vi "decode_image.vi"(4 "width":i32, 6 "heigth":i32, 8 "Color":bool, 9 "M":i32, 10 "max":i16, 11 "Array":u16[](array[numeric])) -> (0 "error out":errorcluster, 3 "image out":T1(plugin-control))   [LabVIEW 2017]
panel:
  out "size(s) 2":i32
  out "size(s)":i32
  out "Array 2":i32[](array[numeric])
  out "x/y 3":dbl
  out "x/y":dbl
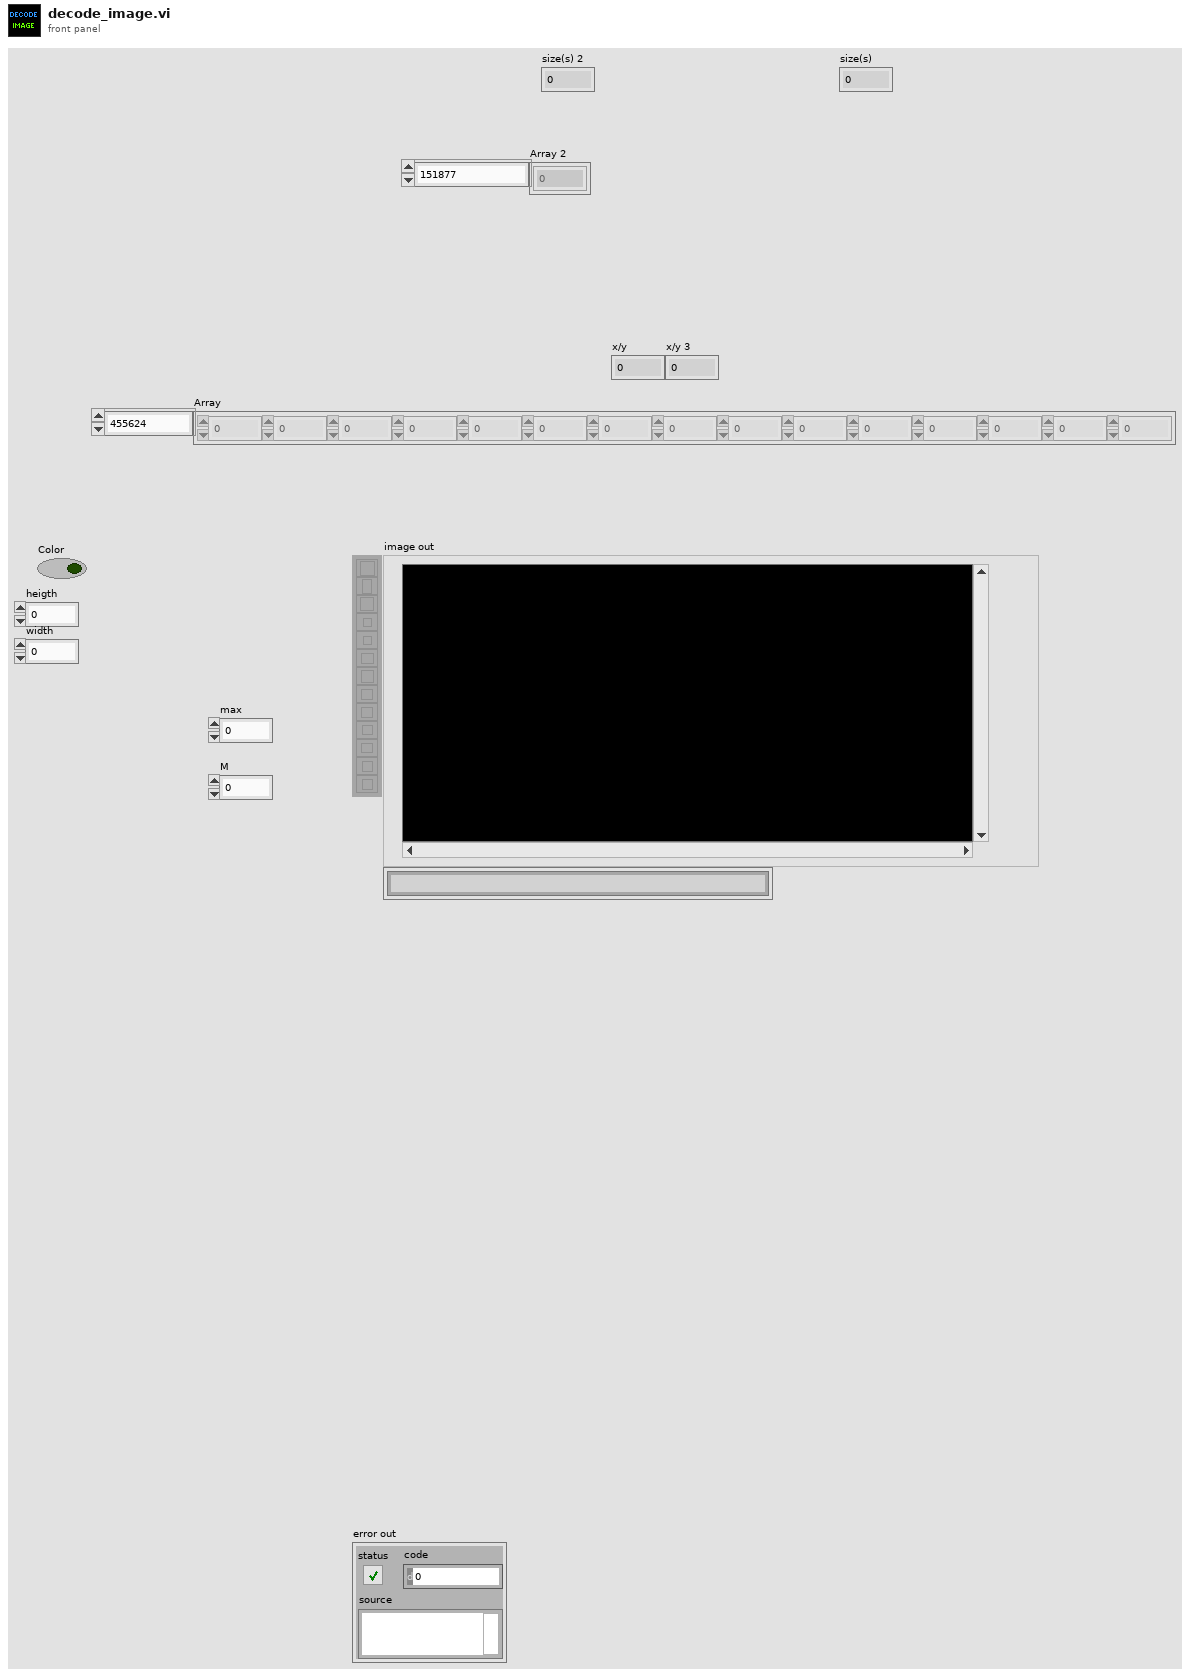
[diagram p1: front panel]
types:
  T1 = typedef "IMAQ Image.ctl" = refnum<image>
  T2 = typedef "Image Type" = u32
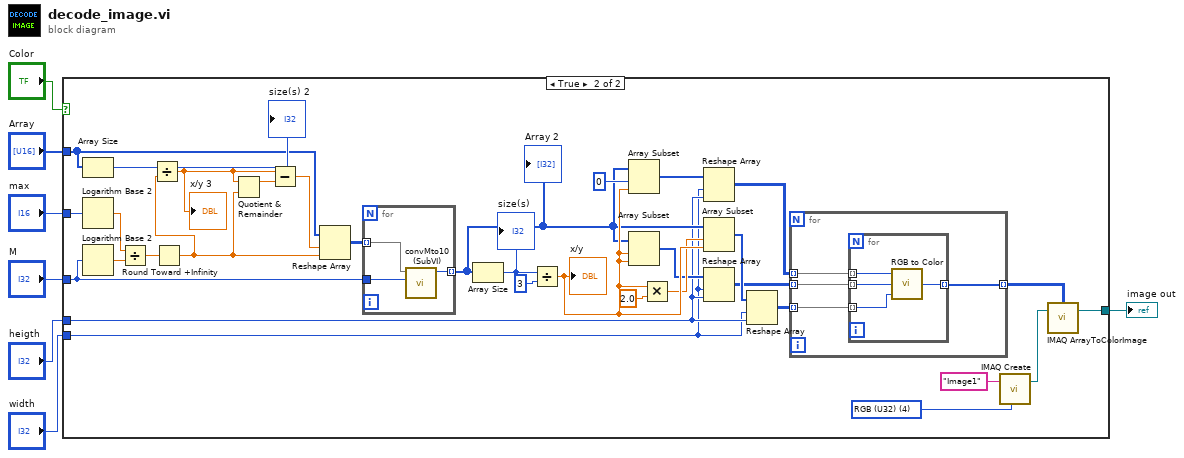
[diagram p0: block diagram]
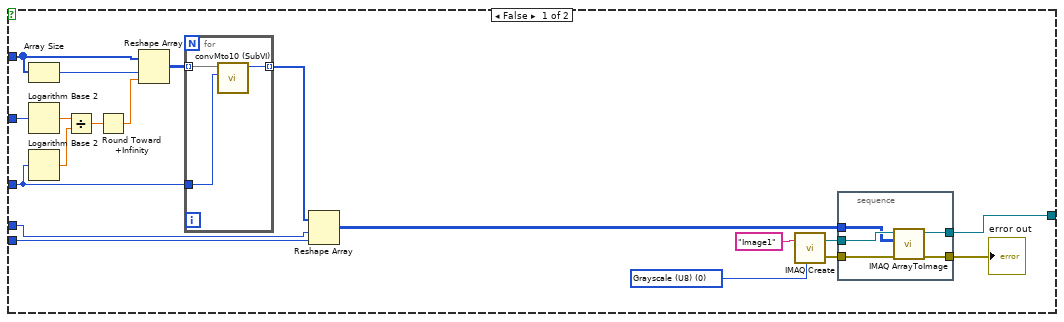
[diagram p2: hidden frame]
diagram:
  n1 = case shown="True" "Color" {
    tunnel: "M" -> [w20 w49]
    tunnel: "Array" -> [w19 w47]
    tunnel: "max" -> [w18 w43]
    tunnel: [w13 w48] -> w4
    tunnel: "heigth" -> [w10 w46]
    tunnel: "width" -> [w9 w45]
    frame False {
      w24 = T2 0 items=["Grayscale (U8)", "Grayscale (I16)", "Grayscale (SGL)", "Complex (CSG)", "RGB (U32)", "HSL (U32)", "RGB (U64)"] ("Image Type")
      n2 = Array Size(array=w19) -> (size(s)=w11:i32)
      n3 = Logarithm Base 2(1:w18) -> (0:w17:dbl)
      n4 = Logarithm Base 2(1:w20) -> (0:w16:dbl)
      n5 = Divide(x=w17, y=w16) -> (x/y=w15:dbl)
      n6 = Round Toward +Infinity(x=w15) -> (ceil(x): smallest int >= x=w14:dbl)
      n7 = Reshape Array(w19, w11, w14) -> (w12:u16[][])
      n8 = for {
        tunnel: w12 -> [w34] mode=indexing
        tunnel: [w33] -> w21 mode=indexing
        tunnel: w20 -> [w32]
        n9 = call "convMto10 (SubVI).vi"("old base"=w32, "value"=w34) -> ("converted value"=w33:i32)  [unwired: 9 in]
      }
      n10 = Reshape Array(w21, w10, w9) -> (w8:i32[][])
      n11 = call "IMAQ Create"("Image Name"="Image1", "Image Type"=w24) -> ("New Image"=w23:T1, "error out"=w26:errorcluster)  [unwired: 3 in]
      n12 = stacked-sequence {
        tunnel: w8 -> [w29]
        tunnel: w23 -> [w31]
        tunnel: [w30] -> w25
        tunnel: w26 -> [w28]
        tunnel: [w27] -> w13
        frame #0 {
          n13 = call "IMAQ ArrayToImage"("error in (no error)"=w28, "Image Pixels (U8)"=w29, "Image"=w31) -> ("error out"=w30:errorcluster, "Image Out"=w27:T1)  [unwired: 7 in]
        }
      }
      "error out" <- w25
    }
    frame True {
      w53 = T2 4 items=["Grayscale (U8)", "Grayscale (I16)", "Grayscale (SGL)", "Complex (CSG)", "RGB (U32)", "HSL (U32)", "RGB (U64)"] ("Image Type")
      n14 = Array Size(array=w47) -> (size(s)=w64:i32)
      "size(s) 2" <- w64
      n15 = Logarithm Base 2(1:w43) -> (0:w65:dbl)
      n16 = Logarithm Base 2(1:w49) -> (0:w66:dbl)
      n17 = Divide(x=w65, y=w66) -> (x/y=w39:dbl)
      n18 = Round Toward +Infinity(x=w39) -> (ceil(x): smallest int >= x=w35:dbl)
      n19 = Divide(x=w64, y=w35) -> (x/y=w37:dbl)
      "x/y 3" <- w37
      n20 = Quotient & Remainder(x=w37, y=w35) -> (x-y*floor(x/y)=w38:dbl)  [unwired: 1 out]
      n21 = Subtract(x=w37, y=w38) -> (x-y=w36:dbl)
      n22 = Reshape Array(w47, w36, w35) -> (w63:u16[][])
      n23 = for {
        tunnel: w63 -> [w77] mode=indexing
        tunnel: w49 -> [w76]
        tunnel: [w75] -> w50 mode=indexing
        n24 = call "convMto10 (SubVI).vi"("old base"=w76, "value"=w77) -> ("converted value"=w75:i32)  [unwired: 9 in]
      }
      "Array 2" <- w50
      n25 = Array Size(array=w50) -> (size(s)=w61:i32)
      "size(s)" <- w61
      n26 = Divide(x=w61, y=3) -> (x/y=w56:dbl)
      "x/y" <- w56
      n27 = Array Subset(array=w50, index=0, length=w56) -> (w62:i32[])
      n28 = Array Subset(array=w50, index=w56, length=w56) -> (w51:i32[])
      n29 = Multiply(x=w56, y=2.0) -> (x*y=w55:dbl)
      n30 = Reshape Array(w62, w45, w46) -> (w42:i32[][])
      n31 = Array Subset(array=w50, index=w55, length=w56) -> (w57:i32[])
      n32 = Reshape Array(w51, w45, w46) -> (w40:i32[][])
      n33 = Reshape Array(w57, w45, w46) -> (w41:i32[][])
      n34 = for {
        tunnel: w42 -> [w70] mode=indexing
        tunnel: [w69] -> w44 mode=indexing
        tunnel: w41 -> [w68] mode=indexing
        tunnel: w40 -> [w67] mode=indexing
        n35 = for {
          tunnel: w70 -> [w74] mode=indexing
          tunnel: [w73] -> w69 mode=indexing
          tunnel: w68 -> [w72] mode=indexing
          tunnel: w67 -> [w71] mode=indexing
          n36 = call <vilib>:"RGB to Color.vi"("B"=w72, "G"=w71, "R"=w74) -> ("Color"=w73:u32)
        }
      }
      n37 = call "IMAQ Create"("Image Name"="Image1", "Image Type"=w53) -> ("New Image"=w52:T1)  [unwired: 3 in, 1 out]
      n38 = call "IMAQ ArrayToColorImage"("Image Pixels (U32)"=w44, "Image"=w52) -> ("Image Out"=w48:T1)  [unwired: 3 in, 1 out]
    }
  }
  "image out" <- w4
